vi "daqio_Refresh_Local_Device.vi"(8 "error in (no error)":errorcluster, 11 "daq.io type in":T6) -> (0 "error out":errorcluster, 1 "found at index":i32, 2 "Dev Types out":T1[](array[typedef]), 3 "daq.io type out":T6, 4 "Dev Type out":T1)   [LabVIEW 2013, in "daqio minimal.lvlib"]
doc: "This VI refreshes the locally stored device information for a specific device by downloading and updating its device type."
uses:
  _typedefs/daqio-Type.ctl
  <vilib>/httpClient/ClientHandle.ctl
  _typedefs/daqio-Device-Type-Info-return.ctl
  _typedefs/daqio-Channel-Type-POST-return.ctl
  _typedefs/daqio-Device.ctl
  _typedefs/daqio-Event-Type.ctl
  _typedefs/daqio-Tag-Type-POST-return.ctl
  _typedefs/FGV_commands.ctl
  daqio minimal.lvlib
  <vilib>/httpClient/LabVIEWHTTPClient.lvlib
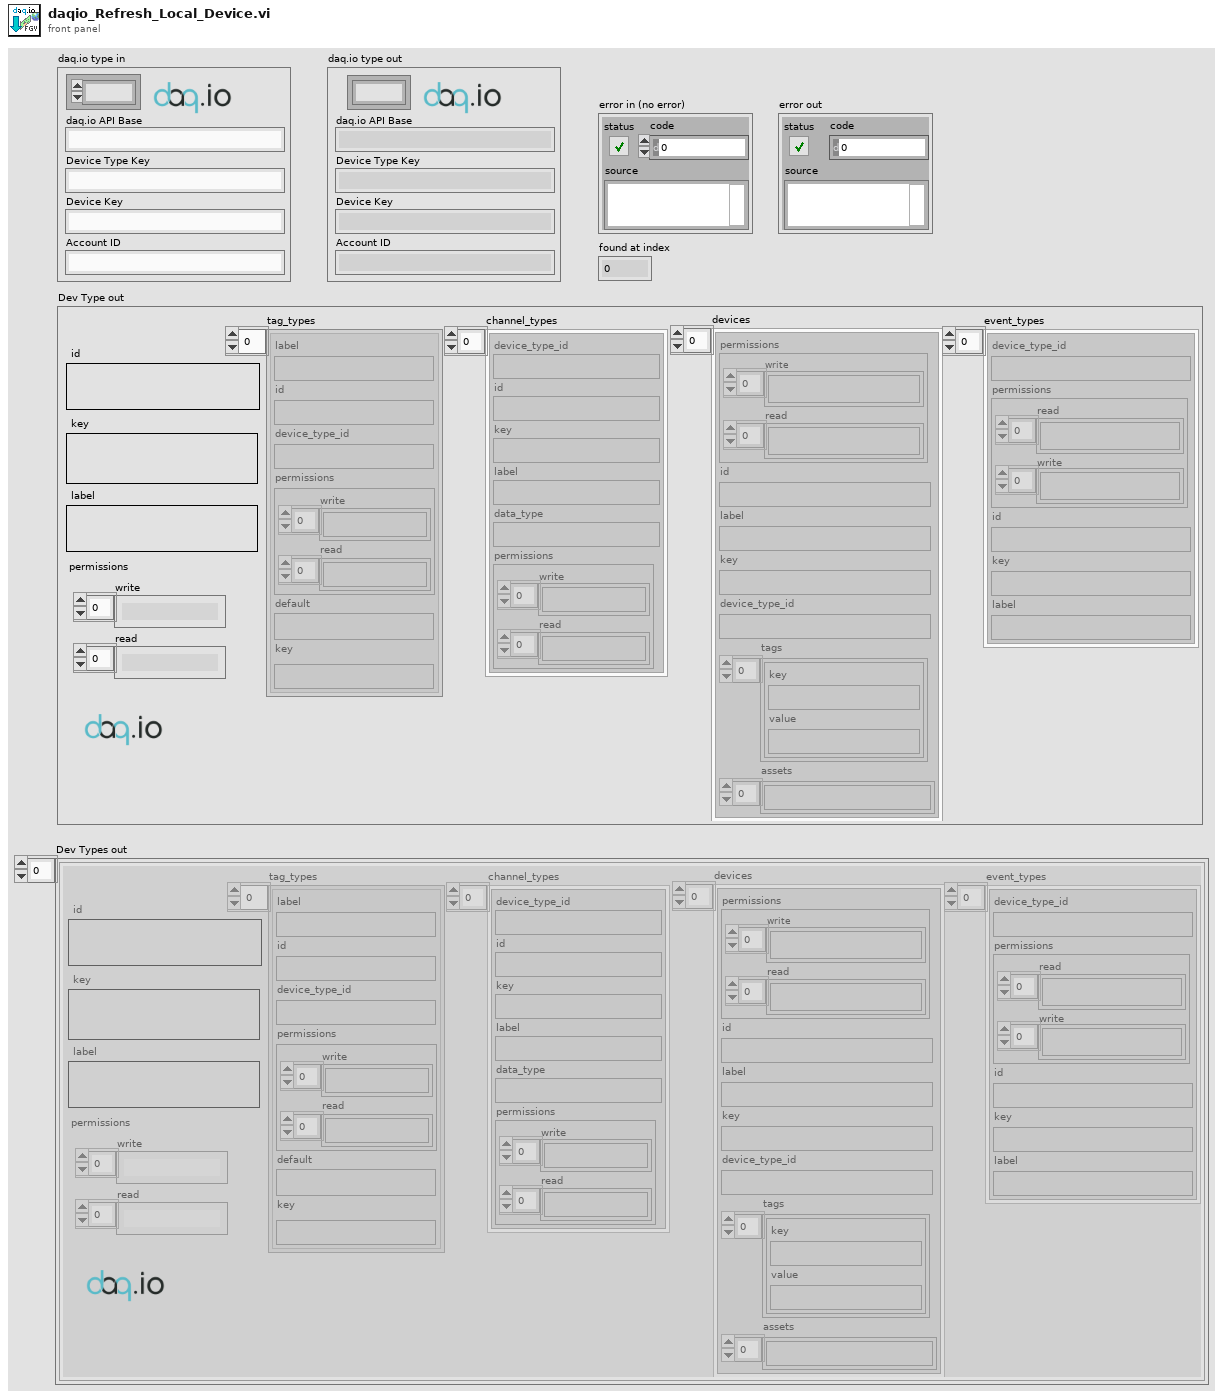
[diagram p1: front panel]
types:
  T1 = typedef "daqio minimal.lvlib/daqio-Device-Type-Info-return.ctl" = cluster{"channel_types":T2[], "devices":T3[], "label":string, "event_types":T4[], "key":string, "tag_types":T5[], "id":string, "permissions":cluster{"write":string[], "read":string[]}}
  T2 = typedef "daqio minimal.lvlib/daqio-Channel-Type-POST-return.ctl" = cluster{"device_type_id":string, "id":string, "key":string, "label":string, "data_type":string, "permissions":cluster{"write":string[], "read":string[]}}
  T3 = typedef "daqio minimal.lvlib/daqio-Device.ctl" = cluster{"permissions":cluster{"write":string[], "read":string[]}, "id":string, "label":string, "key":string, "device_type_id":string, "tags":cluster{"key":string, "value":string}[], "assets":string[]}
  T4 = typedef "daqio minimal.lvlib/daqio-Event-Type.ctl" = cluster{"device_type_id":string, "permissions":cluster{"read":string[], "write":string[]}, "id":string, "key":string, "label":string}
  T5 = typedef "daqio minimal.lvlib/daqio-Tag-Type-POST-return.ctl" = cluster{"label":string, "id":string, "device_type_id":string, "permissions":cluster{"write":string[], "read":string[]}, "default":string, "key":string}
  T6 = typedef "daqio minimal.lvlib/daqio-Type.ctl" = cluster{"daq.io ref":T7, "daq.io API Base":string, "Device Type Key":string, "Device Key":string, "Account ID":string}
  T7 = typedef "LabVIEWHTTPClient.lvlib/ClientHandle.ctl" = refnum<k1>
  T8 = typedef "daqio minimal.lvlib/FGV_commands.ctl" = enum16{"Init / update", "Edit Item", "Find or Add Item", "Remove Item", "Delete All"}
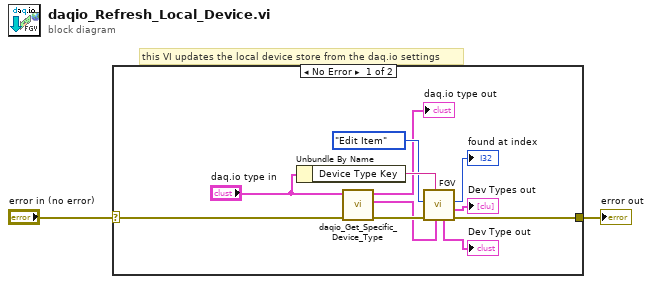
[diagram p0: block diagram]
diagram:
  # "this VI updates the local device store from the daq.io settings"
  n1 = case shown="No Error" "error in (no error)" {
    selector: "error in (no error)" -> [w8 w14]
    tunnel: [w7 w14] -> w1
    frame No Error {
      n2 = Unbundle By Name("daq.io type in") -> ("Device Type Key"=w13:string)
      n3 = call "daqio_Get_Specific_Device_Type.vi"("error in (no error)"=w8, "daq.io type in"="daq.io type in") -> ("error out"=w10:errorcluster, "Device Type"=w6:T1, "daq.io type out"=→"daq.io type out":T6)  [unwired: 7 in]
      n4 = call "FGV.vi"("Dev Type in"=w6, "Dev Type Key"=w13, "error in (no error)"=w10, "Action"=FGV_commands."Edit Item") -> ("error out"=w7:errorcluster, "Dev Types out"=→"Dev Types out":T1[], "found at index"=→"found at index":i32, "Dev Type out"=→"Dev Type out":T1)  [unwired: 3 in, 1 out]
    }
    frame Error {
    }
  }
  "error out" <- w1
